vi "Adjust_Test_Signal_Level.vi"(8 "error in":errorcluster) -> (0 "error out":errorcluster, 2 "OscVoltage":dbl)   [LabVIEW 2020]
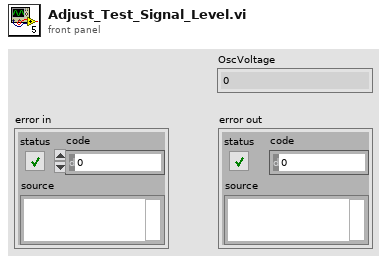
[diagram p1: front panel]
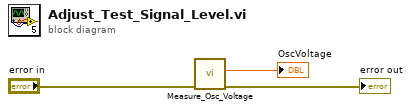
[diagram p0: block diagram]
diagram:
  n1 = call "Measure_Osc_Voltage.vi"("error in"="error in") -> ("error out"=→"error out":errorcluster, "OscVoltage"=→"OscVoltage":dbl)  [unwired: 9 in]
